vi "Inline Wait.vi"(8 "Error In":errorcluster, 11 "milliseconds to wait":u32) -> (0 "Error Out":errorcluster)   [LabVIEW 2017]
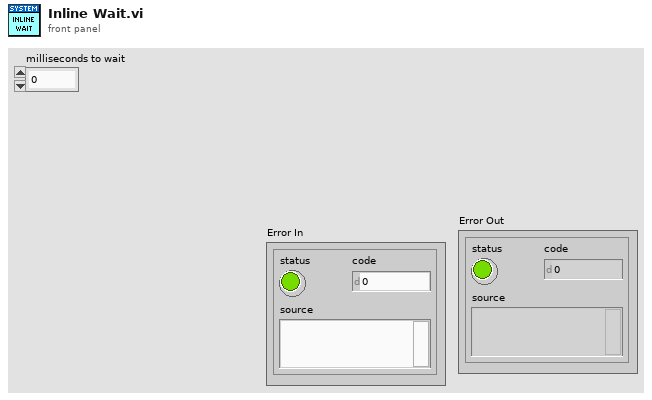
[diagram p1: front panel]
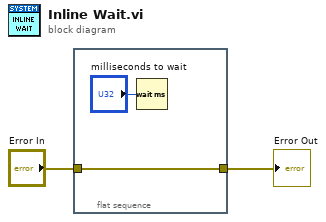
[diagram p0: block diagram]
diagram:
  n1 = flat-sequence {
    tunnel: [w4] -> w2
    tunnel: "Error In" -> [w4]
    frame #0 {
      n2 = Wait (ms)(milliseconds to wait="milliseconds to wait") -> ()  [unwired: 1 out]
    }
  }
  "Error Out" <- w2
